vi "ContourPlot multi-channel v1.vi"() -> ()   [LabVIEW 2020]
uses:
  <vilib>/Utility/file.llb/Read Delimited Spreadsheet (DBL).vi
panel:
  in  "channel index 2":i32=1
  out "Channel number":i32=2
  in  "channel index":i32=2
  in  "Begin":i32
  out "Ready?":bool=TRUE
  in  "Tab Control 2":enum32{"Contour", "Curve"}(tab)
  in  "y index":i32=1
  in  "x index":i32
  out "Intensity Graph":dbl[][](graph)
  in  "Tab Control":enum32{"IV"}(tab)
  out "IV":cluster{dbl[], "Intensity Graph":dbl[]}(graph)
  in  "book number":i32=700
  in  "file path (dialog if empty)":path=path "C:/Users/gyue/Desktop/tmp data folder 20210302"
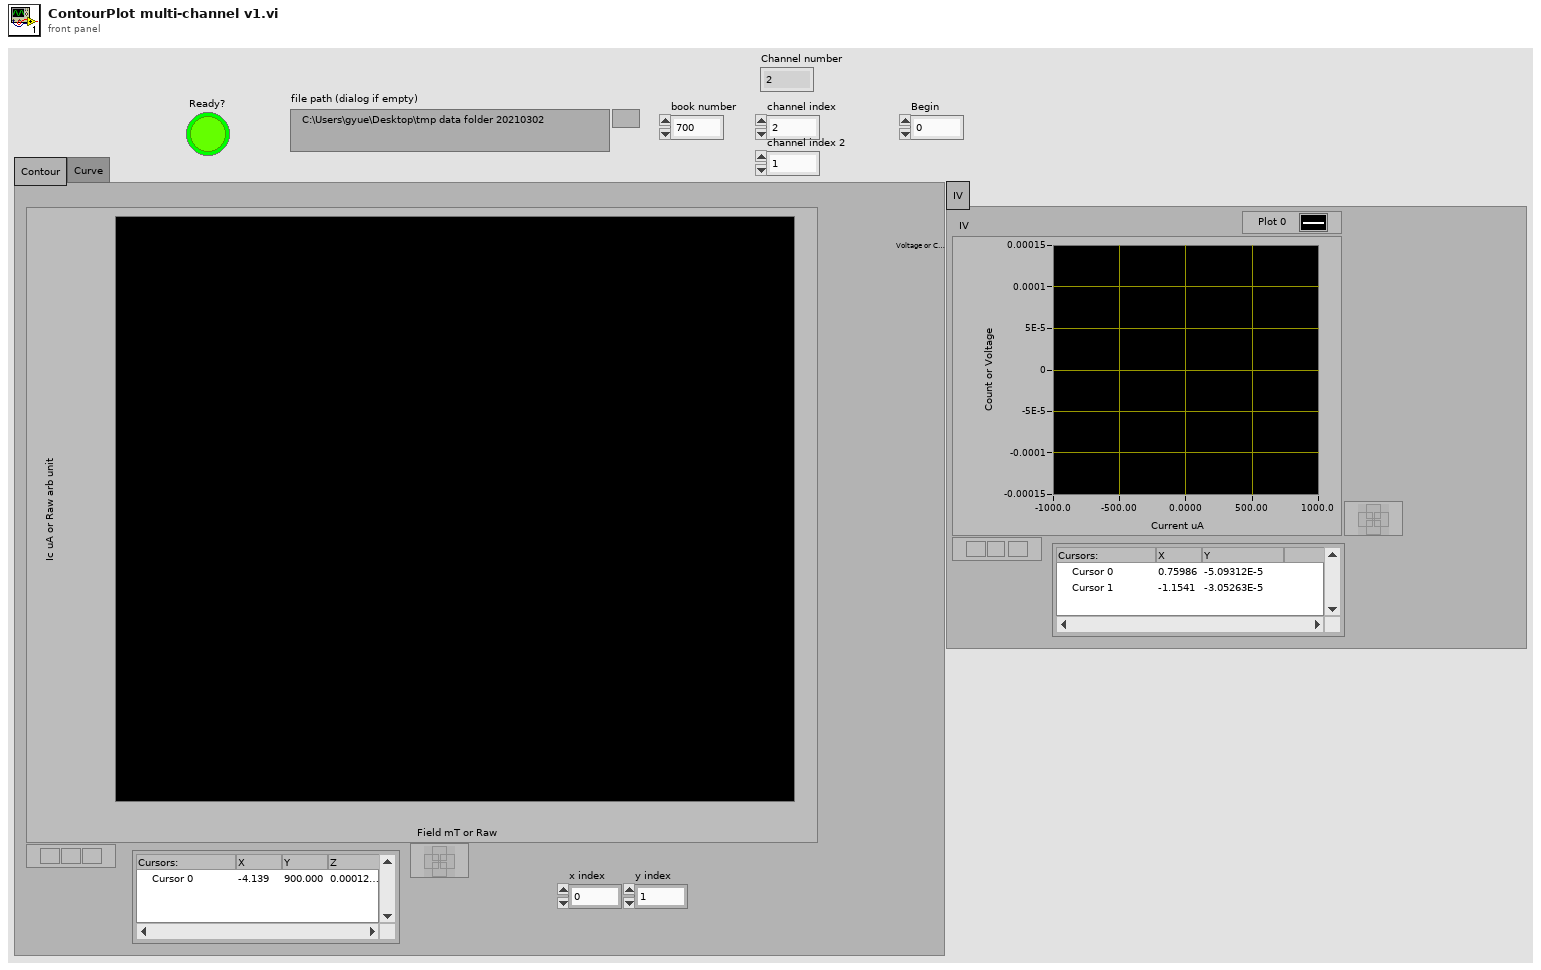
[diagram p1: front panel]
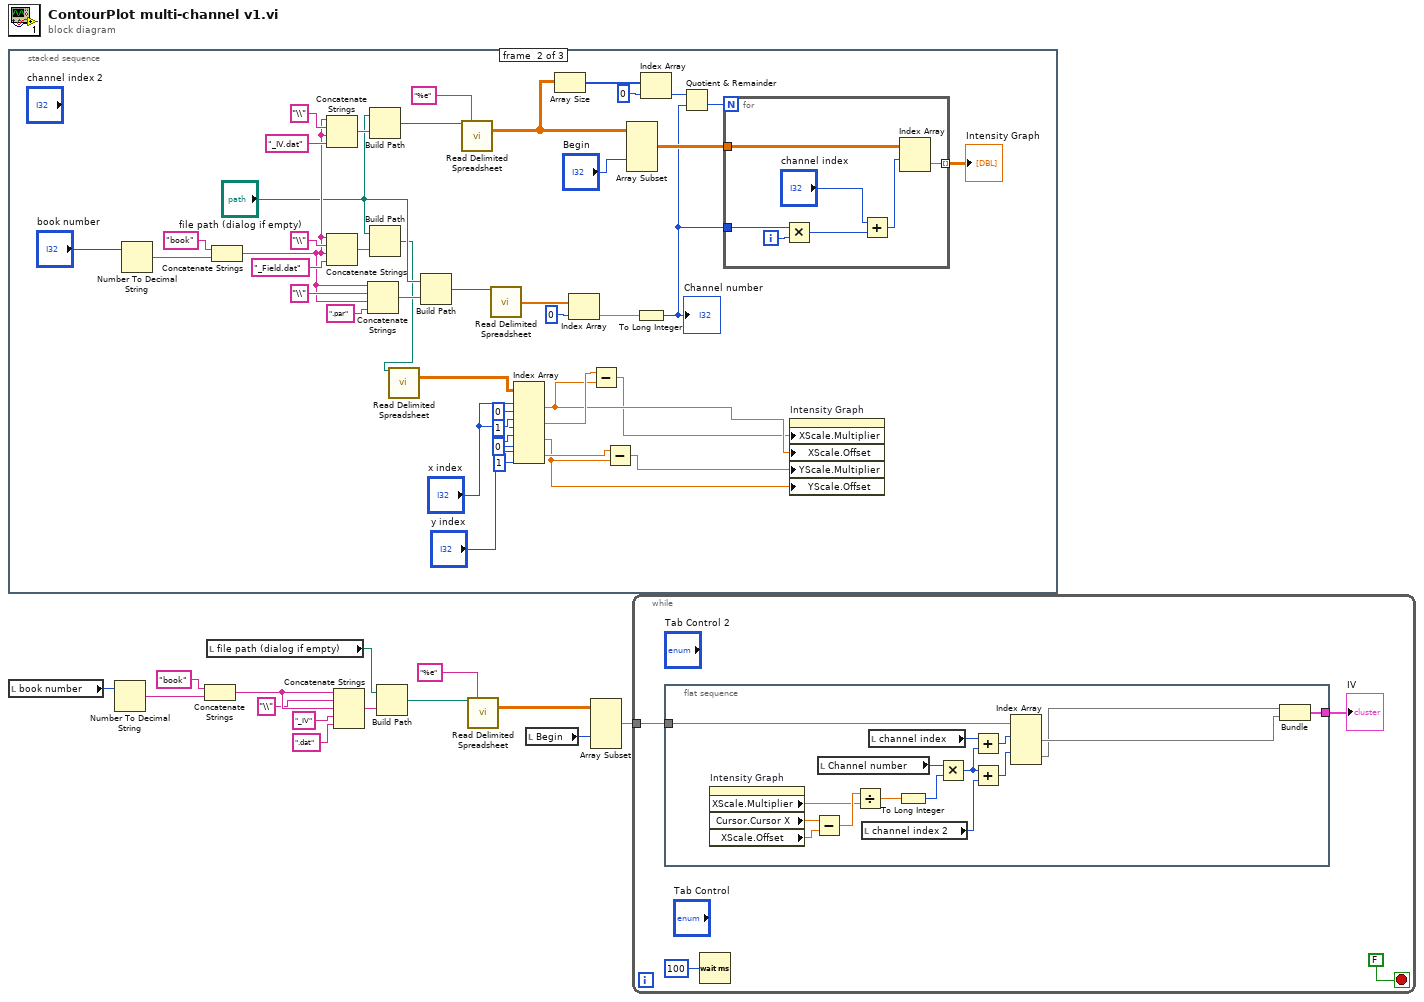
[diagram p0: block diagram]
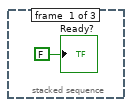
[diagram p2: hidden frame]
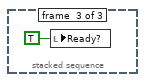
[diagram p3: hidden frame]
diagram:
  n1 = stacked-sequence {
    frame #0 {
      "Ready?" <- FALSE ("Ready?")
    }
    frame #1 {
      n2 = Number To Decimal String(number="book number") -> (decimal integer string=w54:string)  [unwired: 1 in]
      n3 = Concatenate Strings("book" ("string"), w54) -> (w43:string)
      n4 = Concatenate Strings(w43, "\\" ("string"), w43, "_IV.dat" ("string")) -> (w55:string)
      n5 = Concatenate Strings(w43, "\\" ("string"), w43, "_Field.dat" ("string")) -> (w36:string)
      n6 = Concatenate Strings(w43, "\\" ("string"), w43, ".par" ("string")) -> (w56:string)
      n7 = Build Path(base path="file path (dialog if empty)", name or relative path=w55) -> (appended path=w58:path)
      n8 = Build Path(base path="file path (dialog if empty)", name or relative path=w36) -> (appended path=w29:path)
      n9 = call-poly <vilib>:"Read Delimited Spreadsheet.vi"("file path (dialog if empty)"=w29) -> ("all rows"=w28:dbl[][])  [unwired: 9 in, 5 out]
      n10 = Build Path(base path="file path (dialog if empty)", name or relative path=w56) -> (appended path=w57:path)
      n11 = call-poly <vilib>:"Read Delimited Spreadsheet.vi"("file path (dialog if empty)"=w58, "format (%.3f)"="%e") -> ("all rows"=w40:dbl[][])  [unwired: 8 in, 5 out]
      n12 = call-poly <vilib>:"Read Delimited Spreadsheet.vi"("file path (dialog if empty)"=w57) -> ("first row"=w35:dbl[])  [unwired: 9 in, 5 out]
      n13 = Index Array(array=w28, index (row) #1="x index", index (col) #1=0 ("disabled index (col)"), index (row) #2="x index", index (col) #2=1 ("disabled index (col)"), index (row) #3="y index", index (col) #3=0 ("disabled index (col)"), index (row) #4="y index", index (col) #4=1 ("disabled index (col)")) -> (element #1=w23:dbl, element #2=w24:dbl, element #3=w17:dbl, element #4=w18:dbl)
      n14 = Array Size(array=w40) -> (size(s)=w48:i32[])
      n15 = Index Array(array=w35, index=0) -> (element=w33:dbl)
      n16 = Subtract(x=w24, y=w23) -> (x-y=w22:dbl)
      n17 = Subtract(x=w18, y=w17) -> (x-y=w16:dbl)
      n18 = Array Subset(array=w40, index (col)="Begin") -> (w39:dbl[][])  [unwired: 3 in]
      n19 = To Long Integer(number=w33) -> (32bit integer=w31:i32)
      "Channel number" <- w31
      n20 = Index Array(array=w48, index=0) -> (element=w32:i32)
      n21 = Quotient & Remainder(x=w32, y=w31) -> (floor(x/y)=w30:i32)  [unwired: 1 out]
      n22 = for {
        N: w30 -> [_]
        tunnel: w39 -> [w64]
        tunnel: [w63] -> w41 mode=indexing
        tunnel: w31 -> [w60]
        i -> [w65]
        n23 = Multiply(x=w60, y=w65) -> (x*y=w59:i32)
        n24 = Add(x="channel index", y=w59) -> (x+y=w62:i32)
        n25 = Index Array(array=w64, index (row)=w62) -> (element=w63:dbl[])  [unwired: 1 in]
      }
      "Intensity Graph" <- w41
      n26 = property on="Intensity Graph" class="IntGraph (strict)"("XScale.Multiplier"=w22, "XScale.Offset"=w23, "YScale.Multiplier"=w16, "YScale.Offset"=w17) -> ()  [unwired: 2 in, 2 out]
    }
    frame #2 {
      n27 = local write "Ready?"(TRUE ("Ready?")) -> ()
    }
  }
  n28 = local read "book number"() -> (w14:i32)
  n29 = Number To Decimal String(number=w14) -> (decimal integer string=w5:string)  [unwired: 1 in]
  n30 = Concatenate Strings("book" ("string"), w5) -> (w11:string)
  n31 = local read "file path (dialog if empty)"() -> (w4:path)
  n32 = Concatenate Strings(w11, "\\" ("string"), w11, "_IV" ("string"), ".dat" ("string")) -> (w12:string)
  n33 = Build Path(base path=w4, name or relative path=w12) -> (appended path=w13:path)
  n34 = call-poly <vilib>:"Read Delimited Spreadsheet.vi"("file path (dialog if empty)"=w13, "format (%.3f)"="%e") -> ("all rows"=w3:dbl[][])  [unwired: 8 in, 5 out]
  n35 = local read "Begin"() -> (w1:i32)
  n36 = Array Subset(array=w3, index (col)=w1) -> (w2:dbl[][])  [unwired: 3 in]
  n37 = while {
    tunnel: w2 -> [w67]
    stop <- FALSE stop-if-true
    n38 = flat-sequence {
      tunnel: [w82] -> w70
      tunnel: w67 -> [w80]
      frame #0 {
        n39 = property on="Intensity Graph" class="IntGraph (strict)"() -> ("XScale.Multiplier"=w85:dbl, "Cursor.Cursor X"=w84:dbl, "XScale.Offset"=w83:dbl)  [unwired: 2 in, 2 out]
        n40 = Subtract(x=w84, y=w83) -> (x-y=w86:dbl)
        n41 = local read "Channel number"() -> (w78:i32)
        n42 = Divide(x=w86, y=w85) -> (x/y=w81:dbl)
        n43 = local read "channel index 2"() -> (w74:i32)
        n44 = local read "channel index"() -> (w76:i32)
        n45 = To Long Integer(number=w81) -> (32bit integer=w79:i32)
        n46 = Multiply(x=w78, y=w79) -> (x*y=w77:i32)
        n47 = Add(x=w76, y=w77) -> (x+y=w75:i32)
        n48 = Add(x=w77, y=w74) -> (x+y=w73:i32)
        n49 = Index Array(array=w80, index (row) #1=w75, index (row) #2=w73) -> (element #1=w72:dbl[], element #2=w71:dbl[])  [unwired: 2 in]
        n50 = Bundle(w71, w72) -> (w82:cluster{dbl[], dbl[]})  [unwired: 1 in]
      }
    }
    n51 = Wait (ms)(milliseconds to wait=u32 100) -> ()  [unwired: 1 out]
    "IV" <- w70
  }
